vi "Initialize Attributes.vi"(8 "error in (no error)":errorcluster, 10 "Attribute Data":variant, 11 "CS++SVMonitor in":refnum<class "CS++SVMonitor.lvclass">) -> (0 "error out":errorcluster, 2 "Found?":bool, 3 "CS++SVMonitor out":refnum<class "CS++SVMonitor.lvclass">)   [LabVIEW 2012, in "CS++SVMonitor.lvlib" / "CS++SVMonitor.lvclass"]
doc: "Initialize object attribute.\n\nUnique resources should be allocated elsewhere!"
uses:
  CS++SVMonitor.lvclass
  CS++PVMonitor/CS++PVMonitor.lvclass
  CS++SVMonitor.lvclass/CS++SVMonitor.ctl
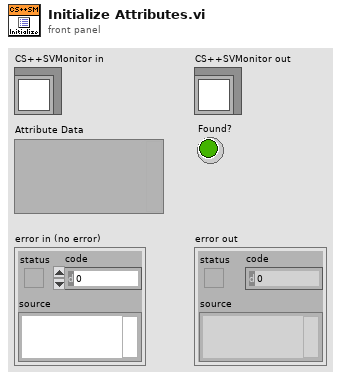
[diagram p1: front panel]
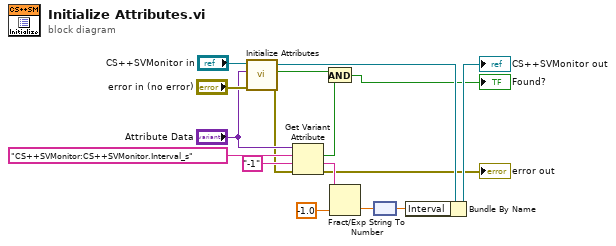
[diagram p0: block diagram]
diagram:
  n1 = call-parent "Initialize Attributes.vi"("error in (no error)"="error in (no error)", "Attribute Data"="Attribute Data", "CS++BaseActor in"="CS++SVMonitor in") -> ("error out"=w2:errorcluster, "Found?"=w16:bool, "CS++BaseActor out"=w6:refnum<class "CS++SVMonitor.lvclass">)  [unwired: 6 in]
  n2 = Get Variant Attribute(Variant="Attribute Data", name="CS++SVMonitor:CS++SVMonitor.Interval_s", default value (empty Variant)="-1", error in=w2) -> (found=w3:bool, value=w10:string, error out=→"error out":errorcluster)  [unwired: 1 out]
  n3 = And(x=w16, y=w3) -> (x .and. y?=→"Found?":bool)
  n4 = Fract/Exp String To Number(string=w10, default (0 dbl)=-1.0) -> (number=w8:dbl)  [unwired: 2 in, 1 out]
  n5 = node(w8) -> (w7:dbl[unit])
  n6 = Bundle By Name(cluster=w6, "Interval"=w7) -> (→"CS++SVMonitor out":refnum<class "CS++SVMonitor.lvclass">)
